vi "Read Single PTU Tag.vi"(8 "error in":errorcluster, 11 "refnum":refnum<file>) -> (0 "error out":errorcluster, 1 "PicoQuant Tag":T1, 3 "refnum out":refnum<file>)   [LabVIEW 2021, in "PTU Files.lvlib"]
uses:
  PTU Files.lvlib
  PicoQuant Header Tag.ctl
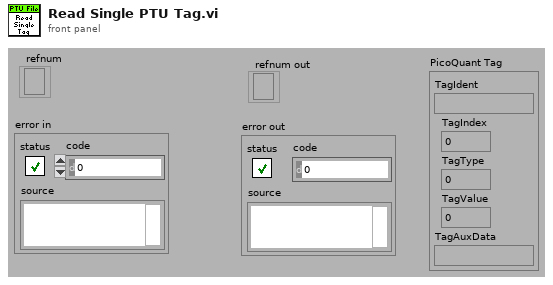
[diagram p1: front panel]
types:
  T1 = typedef "PTU Files.lvlib/PicoQuant Header Tag.ctl" = cluster{"TagIdent":string, "TagIndex":i32, "TagType":i32, "TagValue":i64, "TagAuxData":string}
  T2 = enum16{"big-endian, network order", "native, host order", "little-endian"}
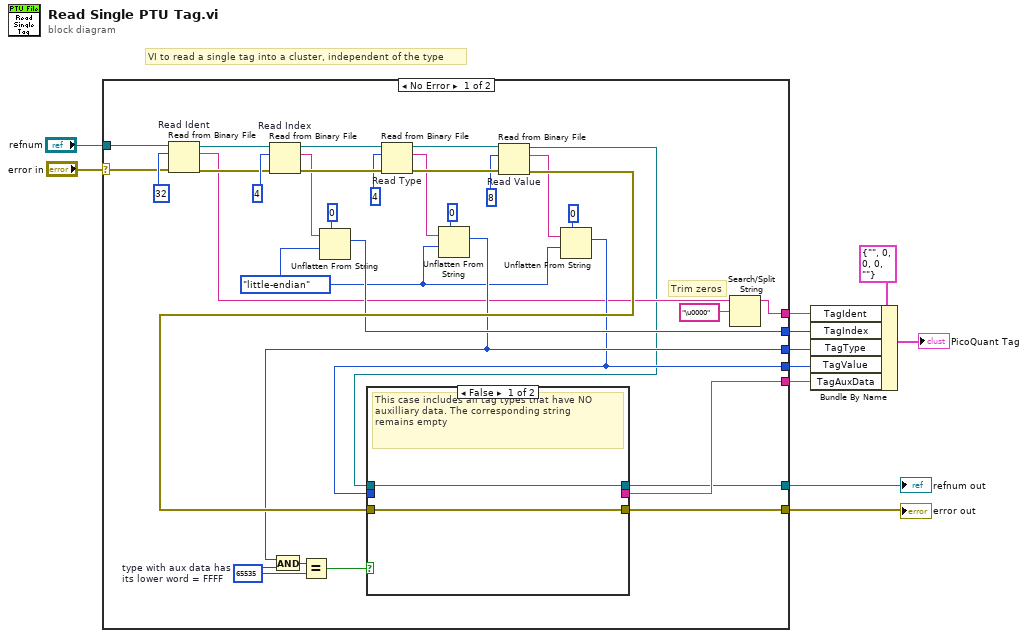
[diagram p0: block diagram]
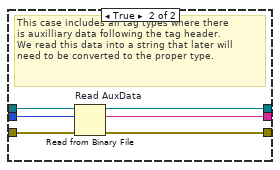
[diagram p2: hidden frame]
diagram:
  # "VI to read a single tag into a cluster, independent of the type"
  n1 = case shown="No Error" "error in" {
    selector: "error in" -> [w29 w54]
    tunnel: "refnum" -> [w14 w53]
    tunnel: [w28 w54] -> w9
    tunnel: [w21 _] -> w4
    tunnel: [w27 _] -> w5
    tunnel: [w26 _] -> w6
    tunnel: [w25 _] -> w7
    tunnel: [w24 _] -> w3
    tunnel: [w13 w53] -> w8
    frame No Error {
      w16 = T2."little-endian" ("byte order (0:big-endian, network order)")
      w32 = 65535  # type with aux data has  its lower word = FFFF
      # "Trim zeros"
      n2 = Read from Binary File "Read Ident"(8:w29, 10:32, 11:w14) -> (0:w30:errorcluster, 2:w22:string, 3:w36:refnum<file>)  [unwired: 3 in, 1 out]
      n3 = Read from Binary File "Read Index"(8:w30, 10:4, 11:w36) -> (0:w40:errorcluster, 2:w17:string, 3:w41:refnum<file>)  [unwired: 3 in, 1 out]
      n4 = Unflatten From String(type=0, binary string=w17, byte order (0:big-endian, network order)=w16) -> (value=w27:i32)  [unwired: 2 in, 2 out]
      n5 = Read from Binary File "Read Type"(8:w40, 10:4, 11:w41) -> (0:w44:errorcluster, 2:w18:string, 3:w43:refnum<file>)  [unwired: 3 in, 1 out]
      n6 = Unflatten From String(type=0, binary string=w18, byte order (0:big-endian, network order)=w16) -> (value=w26:i32)  [unwired: 2 in, 2 out]
      n7 = And(x=w26, y=w32) -> (x .and. y?=w33:i32)
      n8 = Equal?(x=w33, y=w32) -> (x = y?=w12:bool)
      n9 = Read from Binary File "Read Value"(8:w44, 10:8, 11:w43) -> (0:w31:errorcluster, 2:w20:string, 3:w15:refnum<file>)  [unwired: 3 in, 1 out]
      n10 = Unflatten From String(type=i64 0, binary string=w20, byte order (0:big-endian, network order)=w16) -> (value=w25:i64)  [unwired: 2 in, 2 out]
      n11 = case shown="False" w12 {
        tunnel: w25 -> [_ w51]
        tunnel: w15 -> [w45 w50]
        tunnel: w31 -> [w46 w52]
        tunnel: [w46 w49] -> w28
        tunnel: [_ w48] -> w24
        tunnel: [w45 w47] -> w13
        frame False {
          # "This case includes all tag types that have NO \nauxilliary data. The corresponding string \nremains empty"
        }
        frame True {
          # "This case includes all tag types where there \nis auxilliary data following the tag header. \nWe read this data into a string that later will \nneed to be converted to the proper type."
          n12 = Read from Binary File "Read AuxData"(8:w52, 10:w51, 11:w50) -> (0:w49:errorcluster, 2:w48:string, 3:w47:refnum<file>)  [unwired: 3 in, 1 out]
        }
      }
      n13 = Search/Split String(string=w22, search string/char (-)="\u0000" ("string")) -> (substring before match=w21:string)  [unwired: 1 in, 2 out]
    }
    frame Error {
    }
  }
  "error out" <- w9
  "refnum out" <- w8
  n14 = Bundle By Name(cluster=T1 {"TagIdent"="", "TagIndex"=0, "TagType"=0, "TagValue"=0, "TagAuxData"=""} ("PicoQuant Tag"), "TagIdent"=w4, "TagIndex"=w5, "TagType"=w6, "TagValue"=w7, "TagAuxData"=w3) -> (→"PicoQuant Tag":T1)
